vi "Create Path.vi"(8 "error in (no error)":errorcluster) -> (0 "error out":errorcluster, 3 "File Path Control":path)   [LabVIEW 2014, in "Logger.lvlib"]
uses:
  Logger.lvlib
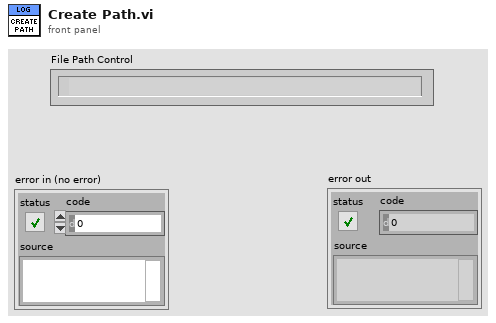
[diagram p1: front panel]
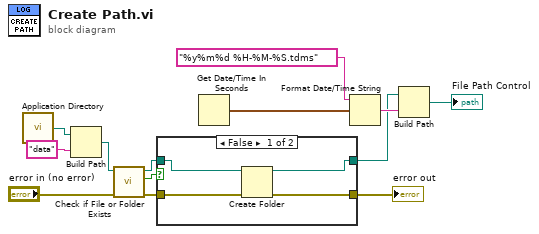
[diagram p0: block diagram]
diagram:
  n1 = call <vilib>:"Application Directory.vi"() -> ("Application Directory"=w13:path)
  n2 = Build Path(base path=w13, name or relative path="data") -> (appended path=w7:path)
  n3 = call <vilib>:"Check if File or Folder Exists.vi"("error in (no error)"="error in (no error)", "path"=w7) -> ("error out"=w3:errorcluster, "file or folder exists?"=w6:bool, "dup path"=w5:path)  [unwired: 7 in]
  n4 = case shown="False" w6 {
    tunnel: w5 -> [w17 w19]
    tunnel: [w14 w19] -> w4
    tunnel: w3 -> [w16 w18]
    tunnel: [w15 w18] -> w1
    frame False {
      n5 = Create Folder(path (use dialog)=w17, error in=w16) -> (created path=w14:path, error out=w15:errorcluster)  [unwired: 1 in, 1 out]
    }
    frame True {
    }
  }
  "error out" <- w1
  n6 = Get Date/Time In Seconds() -> (seconds since 1Jan1904=w11:timestamp)
  n7 = Format Date/Time String(time format string (%c)="%y%m%d %H-%M-%S.tdms", seconds (now)=w11) -> (date/time string=w9:string)  [unwired: 1 in]
  n8 = Build Path(base path=w4, name or relative path=w9) -> (appended path=→"File Path Control":path)
